vi "rsidr_core_global.vi"() -> ()   [LabVIEW 2020, in "Rohde&Schwarz RTx Oscilloscopes.lvlib"] (continued)
is defined by RSRTX_ATTR_HARDCOPY_SELECT_PRINTER attribute. The file name for storage is defined by RSRTX_ATTR_HARDCOPY_FILE_NAME attribute.\n\nAvailable Repeated Capabilities:\nNone\n\nRemote-control command(s):\nHCOPy[:IMMediate]"}, {"Level"=2, "Class Only"=FALSE, "Identifier"="RSRTX_ATTR_HARDCOPY_SELECT_PRINTER", "Descriptive Name"="Hardcopy Select Printer", "Data Type"=2, "Command"="SYST:COMM:PRIN:SEL", "Access"=2, "Range Table"="", "Read Callback"="", "Write Callback"="", "Supported Models"="", "Instrument Options"="", "Flags"=0, "Help"="Selects a configured printer. To determine which printers are installed, use the RSRTX_ATTR_HARDCOPY_GET_FIRST_PRINTER and RSRTX_ATTR_HARDCOPY_GET_NEXT_PRINTER attributes.\n\nAvailable Repeated Capabilities:\nNone\n\nRemote-control command(s):\nSYSTem:COMMunicate:PRINter:SELect"}, {"Level"=2, "Class Only"=FALSE, "Identifier"="RSRTX_ATTR_HARDCOPY_GET_FIRST_PRINTER", "Descriptive Name"="Hardcopy Get First Printer", "Data Type"=2, "Command"="SYST:COMM:PRIN:ENUM:FIRS?", "Access"=0, "Range Table"="", "Read Callback"="", "Write Callback"="", "Supported Models"="", "Instrument Options"="", "Flags"=0, "Help"="Queries the name of the first printer (in the list of printers) available.\nIf no printer is configured an empty string is output.\n\nAvailable Repeated Capabilities:\nNone\n\nRemote-control command(s):\nSYSTem:COMMunicate:PRINter:ENUMerate:FIRSt?"}, {"Level"=2, "Class Only"=FALSE, "Identifier"="RSRTX_ATTR_HARDCOPY_GET_NEXT_PRINTER", "Descriptive Name"="Hardcopy Get Next Printer", "Data Type"=2, "Command"="SYST:COMM:PRIN:ENUM:NEXT?", "Access"=0, "Range Table"="", "Read Callback"="", "Write Callback"="", "Supported Models"="", "Instrument Options"="", "Flags"=0, "Help"="Queries the name of the next printer installed. After all available printer names have been output, an empty string enclosed by quotation marks (&apos;&apos;) is output for the next query. Further queries are answered by a query error.\nThe RSRTX_ATTR_HARDCOPY_GET_FIRST_PRINTER attribute should be sent previously to return to the beginning of the printer list and query the name of the first printer.\n\nAvailable Repeated Capabilities:\nNone\n\nRemote-control command(s):\nSYSTem:COMMunicate:PRINter:ENUMerate[:NEXT]?"}, {"Level"=1, "Class Only"=TRUE, "Identifier"="", "Descriptive Name"="System", "Data Type"=0, "Command"="", "Access"=0, "Range Table"="", "Read Callback"="", "Write Callback"="", "Supported Models"="", "Instrument Options"="", "Flags"=0, "Help"="System attributes."}, {"Level"=2, "Class Only"=FALSE, "Identifier"="RSRTX_ATTR_DEVICE_MODE", "Descriptive Name"="Device Mode", "Data Type"=0, "Command"="DEV:MODE", "Access"=2, "Range Table"="RsRtx_rngDeviceMode", "Read Callback"="", "Write Callback"="", "Supported Models"="", "Instrument Options"="", "Flags"=0, "Help"="Configures the device mode.\n\nAvailable Repeated Capabilities:\nNone\n\nRemote-control command(s):\nDEVice:MODE"}, {"Level"=2, "Class Only"=FALSE, "Identifier"="RSRTX_ATTR_INTERFACE_SELECT", "Descriptive Name"="Interface Select", "Data Type"=0, "Command"="SYST:COMM:INT", "Access"=2, "Range Table"="RsRtx_rngInterface", "Read Callback"="", "Write Callback"="", "Supported Models"="", "Instrument Options"="", "Flags"=0, "Help"="Selects the interface for remote control and web browser access ( ETHernet only).\n\nAvailable Repeated Capabilities:\nNone\n\nRemote-control command(s):\nSYSTem:COMMunicate:INTerface[:SELect]"}, {"Level"=2, "Class Only"=FALSE, "Identifier"="RSRTX_ATTR_USB_CLASS", "Descriptive Name"="USB Class", "Data Type"=0, "Command"="SYST:COMM:INT:USB:CLAS", "Access"=2, "Range Table"="RsRtx_rngUSBClass", "Read Callback"="", "Write Callback"="", "Supported Models"="", "Instrument Options"="", "Flags"=0, "Help"="Selects the USB mode.\n\nAvailable Repeated Capabilities:\nNone\n\nRemote-control command(s):\nSYSTem:COMMunicate:INTerface:USB:CLASs"}, {"Level"=2, "Class Only"=FALSE, "Identifier"="RSRTX_ATTR_ETHERNET_DHCP", "Descriptive Name"="Ethernet DHCP", "Data Type"=3, "Command"="SYST:COMM:INT:ETH:DHCP", "Access"=2, "Range Table"="", "Read Callback"="", "Write Callback"="", "Supported Models"="", "Instrument Options"="", "Flags"=0, "Help"="Enables DHCP for automatic network parameter distribution.\n\nAvailable Repeated Capabilities:\nNone\n\nRemote-control command(s):\nSYSTem:COMMunicate:INTerface:ETHernet:DHCP"}, {"Level"=2, "Class Only"=FALSE, "Identifier"="RSRTX_ATTR_ETHERNET_IP_PORT", "Descriptive Name"="Ethernet IP Port", "Data Type"=0, "Command"="SYST:COMM:INT:ETH:IPP", "Access"=2, "Range Table"="RsRtx_rngEthernetIPPort", "Read Callback"="", "Write Callback"="", "Supported Models"="", "Instrument Options"="", "Flags"=0, "Help"="Specify the IP port number.\n\nAvailable Repeated Capabilities:\nNone\n\nRemote-control command(s):\nSYSTem:COMMunicate:INTerface:ETHernet:IPPort"}, {"Level"=2, "Class Only"=FALSE, "Identifier"="RSRTX_ATTR_ETHERNET_VXI11_PORT", "Descriptive Name"="Ethernet VXI11 Port", "Data Type"=0, "Command"="SYST:COMM:INT:ETH:VXIP", "Access"=2, "Range Table"="RsRtx_rng16BitRange", "Read Callback"="", "Write Callback"="", "Supported Models"="", "Instrument Options"="", "Flags"=0, "Help"="Returns or specifies the VXI-11 port number.\n\nAvailable Repeated Capabilities:\nNone\n\nRemote-control command(s):\nSYSTem:COMMunicate:INTerface:ETHernet:VXIPort"}, {"Level"=2, "Class Only"=FALSE, "Identifier"="RSRTX_ATTR_ETHERNET_HTTP_PORT", "Descriptive Name"="Ethernet HTTP Port", "Data Type"=0, "Command"="SYST:COMM:INT:ETH:HTTP", "Access"=2, "Range Table"="RsRtx_rng16BitRange", "Read Callback"="", "Write Callback"="", "Supported Models"="", "Instrument Options"="", "Flags"=0, "Help"="Returns or specifies the HTTP port number.\n\nAvailable Repeated Capabilities:\nNone\n\nRemote-control command(s):\nSYSTem:COMMunicate:INTerface:ETHernet:HTTPport"}, {"Level"=2, "Class Only"=FALSE, "Identifier"="RSRTX_ATTR_ETHERNET_TRANSFER", "Descriptive Name"="Ethernet Transfer", "Data Type"=0, "Command"="SYST:COMM:INT:ETH:TRAN", "Access"=2, "Range Table"="RsRtx_rngEthernetTransfer", "Read Callback"="", "Write Callback"="", "Supported Models"="", "Instrument Options"="", "Flags"=0, "Help"="Enables automatic transfer speed selection, or selects one of the predefined settings that corresponds to your network data rate.\n\nAvailable Repeated Capabilities:\nNone\n\nRemote-control command(s):\nSYSTem:COMMunicate:INTerface:ETHernet:TRANsfer"}, {"Level"=2, "Class Only"=FALSE, "Identifier"="RSRTX_ATTR_ETHERNET_MAC_ADDRESS", "Descriptive Name"="Ethernet MAC Address", "Data Type"=2, "Command"="SYST:COMM:INT:ETH:MAC?", "Access"=0, "Range Table"="", "Read Callback"="", "Write Callback"="", "Supported Models"="", "Instrument Options"="", "Flags"=0, "Help"="Returns the instrument&apos;s media access control address.\n\nAvailable Repeated Capabilities:\nNone\n\nRemote-control command(s):\nSYSTem:COMMunicate:INTerface:ETHernet:MACaddress?"}, {"Level"=2, "Class Only"=FALSE, "Identifier"="RSRTX_ATTR_PRESET_EDUCATION", "Descriptive Name"="Preset Education", "Data Type"=4, "Command"="SYST:EDUC:PRES", "Access"=1, "Range Table"="", "Read Callback"="", "Write Callback"="", "Supported Models"="", "Instrument Options"="", "Flags"=0, "Help"="Deletes the password of the education mode.\n\nAvailable Repeated Capabilities:\nNone\n\nRemote-control command(s):\nSYSTem:EDUCation:PRESet"}, {"Level"=2, "Class Only"=FALSE, "Identifier"="RSRTX_ATTR_DEVICE_FOOTPRINT", "Descriptive Name"="Device Footprint", "Data Type"=2, "Command"="SYST:DFPR?", "Access"=0, "Range Table"="", "Read Callback"="", "Write Callback"="", "Supported Models"="", "Instrument Options"="", "Flags"=0, "Help"="Returns the device footprint of the instrument. The device footprint contains the configuration of the instrument, installed modules, installed software and software licenses. This information is written in the device footprint xml file might be useful in case of maintenance or support request.\n\nAvailable Repeated Capabilities:\nNone\n\nRemote-control command(s):\nSYSTem:DFPRint?"}, {"Level"=1, "Class Only"=TRUE, "Identifier"="", "Descriptive Name"="Utility Functions", "Data Type"=0, "Command"="", "Access"=0, "Range Table"="", "Read Callback"="", "Write Callback"="", "Supported Models"="", "Instrument Options"="", "Flags"=0, "Help"="This subsystem contains functions for Utility Functions."}, {"Level"=2, "Class Only"=FALSE, "Identifier"="RSRTX_ATTR_SYSTEM_PRESET", "Descriptive Name"="System Preset", "Data Type"=4, "Command"="SYST:PRES", "Access"=1, "Range Table"="", "Read Callback"="", "Write Callback"="", "Supported Models"="", "Instrument Options"="", "Flags"=0, "Help"="Presets all parameters.\n\nAvailable Repeated Capabilities:\nNone\n\nRemote-control command(s):\nSYSTem:PRESet"}, {"Level"=2, "Class Only"=FALSE, "Identifier"="RSRTX_ATTR_CALIBRATION", "Descriptive Name"="Calibration", "Data Type"=0, "Command"="*CAL?", "Access"=0, "Range Table"="", "Read Callback"="", "Write Callback"="", "Supported Models"="", "Instrument Options"="", "Flags"=0, "Help"="Initiates a calibration of the instrument and subsequently queries the calibration status. Responses > 0 indicate errors.\n\nAvailable Repeated Capabilities:\nNone\n\nRemote-control command(s):\n*CAL?"}, {"Level"=2, "Class Only"=FALSE, "Identifier"="RSRTX_ATTR_SELF_TEST_QUERY", "Descriptive Name"="Self-Test Query", "Data Type"=0, "Command"="*TST?", "Access"=0, "Range Table"="", "Read Callback"="", "Write Callback"="", "Supported Models"="", "Instrument Options"="", "Flags"=1, "Help"="Triggers selftests of the instrument and returns an error code in decimal form (see Service Manual supplied with the instrument). 0 indicates no errors occured.\n\nAvailable Repeated Capabilities:\nNone\n\nRemote-control command(s):\n*TST?"}, {"Level"=2, "Class Only"=FALSE, "Identifier"="RSRTX_ATTR_SYSTEM_ERROR", "Descriptive Name"="System Error", "Data Type"=2, "Command"="SYST:ERR?", "Access"=0, "Range Table"="", "Read Callback"="", "Write Callback"="", "Supported Models"="", "Instrument Options"="", "Flags"=0, "Help"="Queries error from error queue.\n\nAvailable Repeated Capabilities:\nNone\n\nRemote-control command(s):\nSYSTem:ERRor:[NEXT]?"}, {"Level"=2, "Class Only"=FALSE, "Identifier"="RSRTX_ATTR_SYST_ERR_LIST", "Descriptive Name"="System Error List", "Data Type"=2, "Command"="SYST:ERR:ALL?", "Access"=0, "Range Table"="", "Read Callback"="", "Write Callback"="", "Supported Models"="", "Instrument Options"="", "Flags"=0, "Help"="Returns the error message string read from the instrument&apos;s error message queue.\n\nAvailable Repeated Capabilities:\nNone\n\nRemote-control command(s):\nSYSTem:ERRor:ALL?"}, {"Level"=2, "Class Only"=FALSE, "Identifier"="RSRTX_ATTR_INSTRUMENT_NAME", "Descriptive Name"="Instrument Name", "Data Type"=2, "Command"="SYST:NAME", "Access"=2, "Range Table"="", "Read Callback"="", "Write Callback"="", "Supported Models"="", "Instrument Options"="", "Flags"=0, "Help"="Defines an instrument name (String with max. 20 characters).\n\nAvailable Repeated Capabilities:\nNone\n\nRemote-control command(s):\nSYSTem:NAME"}, {"Level"=2, "Class Only"=FALSE, "Identifier"="RSRTX_ATTR_RESET_STATUS_REGISTER", "Descriptive Name"="Reset Status Register", "Data Type"=4, "Command"="STAT:PRES", "Access"=1, "Range Table"="", "Read Callback"="", "Write Callback"="", "Supported Models"="", "Instrument Options"="", "Flags"=0, "Help"="Resets all STATUS:QUESTIONALBLE registers.\n\nAvailable Repeated Capabilities:\nNone\n\nRemote-control command(s):\nSTATus:PRESet"}, {"Level"=2, "Class Only"=FALSE, "Identifier"="RSRTX_ATTR_SELF_ALIGNMENT", "Descriptive Name"="Self Alignment", "Data Type"=4, "Command"="CAL", "Access"=1, "Range Table"="", "Read Callback"="", "Write Callback"="", "Supported Models"="", "Instrument Options"="", "Flags"=0, "Help"="Executes an internal self-alignment of the instrument.\n\nAvailable Repeated Capabilities:\nNone\n\nRemote-control command(s):\nCALibration"}, {"Level"=2, "Class Only"=FALSE, "Identifier"="RSRTX_ATTR_SELF_ALIGNMENT_STATE", "Descriptive Name"="Self Alignment State", "Data Type"=0, "Command"="CAL:STAT?", "Access"=0, "Range Table"="rsrtx_rngSelfAlignmentState", "Read Callback"="", "Write Callback"="", "Supported Models"="", "Instrument Options"="", "Flags"=0, "Help"="Returns the overall state of the self-alignment.\n\nAvailable Repeated Capabilities:\nNone\n\nRemote-control command(s):\nCALibration:STATe?"}, {"Level"=2, "Class Only"=FALSE, "Identifier"="RSRTX_ATTR_QUERY_OPC", "Descriptive Name"="Query OPC", "Data Type"=0, "Command"="*OPC?", "Access"=0, "Range Table"="", "Read Callback"="", "Write Callback"="", "Supported Models"="", "Instrument Options"="", "Flags"=0, "Help"="Queries the OPC.\n\nAvailable Repeated Capabilities:\nNone\n\nRemote-control command(s):\n*OPC?"}, {"Level"=2, "Class Only"=FALSE, "Identifier"="RSRTX_ATTR_PROCESS_ALL_PREVIOUS_COMMANDS", "Descriptive Name"="Process All Previous Commands", "Data Type"=4, "Command"="*WAI", "Access"=1, "Range Table"="", "Read Callback"="", "Write Callback"="", "Supported Models"="", "Instrument Options"="", "Flags"=2, "Help"="Stops further command processing until all commands sent before *WAI have been executed.\n\nAvailable Repeated Capabilities:\nNone\n\nRemote-control command(s):\n*WAI"}, {"Level"=2, "Class Only"=TRUE, "Identifier"="", "Descriptive Name"="Sound", "Data Type"=0, "Command"="", "Access"=0, "Range Table"="", "Read Callback"="", "Write Callback"="", "Supported Models"="", "Instrument Options"="", "Flags"=0, "Help"="Additional Sound Attributes."}, {"Level"=3, "Class Only"=FALSE, "Identifier"="RSRTX_ATTR_SOUND_ENABLED", "Descriptive Name"="Sound Enabled", "Data Type"=3, "Command"="SYST:BEEP:CONT:STAT", "Access"=2, "Range Table"="", "Read Callback"="", "Write Callback"="", "Supported Models"="", "Instrument Options"="", "Flags"=0, "Help"="Enables or diables a sound for general control events, e.g. reaching the rotary encoder end or changing the measuring mode in the Automeasure menu.\n\nAvailable Repeated Capabilities:\nNone\n\nRemote-control command(s):\nSYSTem:BEEPer:CONTrol:STATe"}, {"Level"=3, "Class Only"=FALSE, "Identifier"="RSRTX_ATTR_SOUND_ERROR_ENABLED", "Descriptive Name"="Sound Error Enabled", "Data Type"=3, "Command"="SYST:BEEP:ERR:STAT", "Access"=2, "Range Table"="", "Read Callback"="", "Write Callback"="", "Supported Models"="", "Instrument Options"="", "Flags"=0, "Help"="Enables or disables the beep if an error occurs.\n\nAvailable Repeated Capabilities:\nNone\n\nRemote-control command(s):\nSYSTem:BEEPer:ERRor:STATe"}, {"Level"=3, "Class Only"=FALSE, "Identifier"="RSRTX_ATTR_SOUND_TRIGGER_ENABLED", "Descriptive Name"="Sound Trigger Enabled", "Data Type"=3, "Command"="SYST:BEEP:TRIG:STAT", "Access"=2, "Range Table"="", "Read Callback"="", "Write Callback"="", "Supported Models"="", "Instrument Options"="", "Flags"=0, "Help"="Enables or disables the beep if a trigger occurs.\n\nAvailable Repeated Capabilities:\nNone\n\nRemote-control command(s):\nSYSTem:BEEPer:TRIG:STATe"}, {"Level"=3, "Class Only"=FALSE, "Identifier"="RSRTX_ATTR_SOUND_GENERATE", "Descriptive Name"="Sound Generate", "Data Type"=4, "Command"="SYST:BEEP", "Access"=1, "Range Table"="", "Read Callback"="", "Write Callback"="", "Supported Models"="", "Instrument Options"="", "Flags"=0, "Help"="Generates an immediate beep.\n\nAvailable Repeated Capabilities:\nNone\n\nRemote-control command(s):\nSYSTem:BEEPer[:IMMediate]"}, {"Level"=2, "Class Only"=TRUE, "Identifier"="", "Descriptive Name"="Status Register", "Data Type"=0, "Command"="", "Access"=0, "Range Table"="", "Read Callback"="", "Write Callback"="", "Supported Models"="", "Instrument Options"="", "Flags"=0, "Help"="Configures the status reporting system."}, {"Level"=3, "Class Only"=TRUE, "Identifier"="", "Descriptive Name"="Operation", "Data Type"=0, "Command"="", "Access"=0, "Range Table"="", "Read Callback"="", "Write Callback"="", "Supported Models"="", "Instrument Options"="", "Flags"=0, "Help"="Configures the operation status reporting system."}, {"Level"=4, "Class Only"=FALSE, "Identifier"="RSRTX_ATTR_OPERATION_CONDITION", "Descriptive Name"="Operation Condition", "Data Type"=0, "Command"="STAT:OPER:COND?", "Access"=0, "Range Table"="", "Read Callback"="", "Write Callback"="", "Supported Models"="", "Instrument Options"="", "Flags"=0, "Help"="Sets the status reporting system Operation Condition.\n\nNote:\n(1) For detailed description of Status Reporting System see also operating manual.\n\nAvailable Repeated Capabilities:\nNone\n\nRemote-control command(s):\nSTATus:OPERation:CONDition?"}, {"Level"=4, "Class Only"=FALSE, "Identifier"="RSRTX_ATTR_OPERATION_ENABLE", "Descriptive Name"="Operation Enable", "Data Type"=0, "Command"="STAT:OPER:ENAB", "Access"=2, "Range Table"="", "Read Callback"="", "Write Callback"="", "Supported Models"="", "Instrument Options"="", "Flags"=0, "Help"="Sets the status reporting system Operation Enable.\n\nNote:\n(1) For detailed description of Status Reporting System see also operating manual.\n\nAvailable Repeated Capabilities:\nNone\n\nRemote-control command(s):\nSTATus:OPERation:ENABle"}, {"Level"=4, "Class Only"=FALSE, "Identifier"="RSRTX_ATTR_OPERATION_N_TRANSITION", "Descriptive Name"="Operation N Transition", "Data Type"=0, "Command"="STAT:OPER:NTR", "Access"=2, "Range Table"="", "Read Callback"="", "Write Callback"="", "Supported Models"="", "Instrument Options"="", "Flags"=0, "Help"="Sets the status reporting system Operation N Transition.\n\nNote:\n(1) For detailed description of Status Reporting System see also operating manual.\n\nAvailable Repeated Capabilities:\nNone\n\nRemote-control command(s):\nSTATus:OPERation:NTRansition"}, {"Level"=4, "Class Only"=FALSE, "Identifier"="RSRTX_ATTR_OPERATION_P_TRANSITION", "Descriptive Name"="Operation P Transition", "Data Type"=0, "Command"="STAT:OPER:PTR", "Access"=2, "Range Table"="", "Read Callback"="", "Write Callback"="", "Supported Models"="", "Instrument Options"="", "Flags"=0, "Help"="Sets the status reporting system Operation P Transition.\n\nNote:\n(1) For detailed description of Status Reporting System see also operating manual.\n\nAvailable Repeated Capabilities:\nNone\n\nRemote-control command(s):\nSTATus:OPERation:PTRansition"}, {"Level"=4, "Class Only"=FALSE, "Identifier"="RSRTX_ATTR_OPERATION_EVENT", "Descriptive Name"="Operation Event", "Data Type"=0, "Command"="STAT:OPER?", "Access"=0, "Range Table"="", "Read Callback"="", "Write Callback"="", "Supported Models"="", "Instrument Options"="", "Flags"=0, "Help"="Sets the status reporting system Operation Event.\n\nNote:\n(1) For detailed description of Status Reporting System see also operating manual.\n\nAvailable Repeated Capabilities:\nNone\n\nRemote-control command(s):\nSTATus:OPERation[:EVENt]?"}, {"Level"=3, "Class Only"=TRUE, "Identifier"="", "Descriptive Name"="Questionable", "Data Type"=0, "Command"="", "Access"=0, "Range Table"="", "Read Callback"="", "Write Callback"="", "Supported Models"="", "Instrument Options"="", "Flags"=0, "Help"="Configures the questionable status reporting system."}, {"Level"=4, "Class Only"=FALSE, "Identifier"="RSRTX_ATTR_QUESTIONABLE_CONDITION", "Descriptive Name"="Questionable Condition", "Data Type"=0, "Command"="STAT:QUES:COND?", "Access"=0, "Range Table"="RsRtx_rng16BitRange", "Read Callback"="", "Write Callback"="", "Supported Models"="", "Instrument Options"="", "Flags"=0, "Help"="Sets the status reporting system Questionable Condition.\n\nNote:\n(1) For detailed description of Status Reporting System see also operating manual.\n\nAvailable Repeated Capabilities:\nNone\n\nRemote-control command(s):\nSTATus:QUEStionable:CONDition?"}, {"Level"=4, "Class Only"=FALSE, "Identifier"="RSRTX_ATTR_QUESTIONABLE_ENABLE", "Descriptive Name"="Questionable Enable", "Data Type"=0, "Command"="STAT:QUES:ENAB", "Access"=2, "Range Table"="RsRtx_rng16BitRange", "Read Callback"="", "Write Callback"="", "Supported Models"="", "Instrument Options"="", "Flags"=0, "Help"="Sets the status reporting system Questionable Enable.\n\nNote:\n(1) For detailed description of Status Reporting System see also operating manual.\n\nAvailable Repeated Capabilities:\nNone\n\nRemote-control command(s):\nSTATus:QUEStionable:ENABle"}, {"Level"=4, "Class Only"=FALSE, "Identifier"="RSRTX_ATTR_QUESTIONABLE_N_TRANSITION", "Descriptive Name"="Questionable N Transition", "Data Type"=0, "Command"="STAT:QUES:NTR", "Access"=2, "Range Table"="RsRtx_rng16BitRange", "Read Callback"="", "Write Callback"="", "Supported Models"="", "Instrument Options"="", "Flags"=0, "Help"="Sets the status reporting system Questionable N Transition.\n\nNote:\n(1) For detailed description of Status Reporting System see also operating manual.\n\nAvailable Repeated Capabilities:\nNone\n\nRemote-control command(s):\nSTATus:QUEStionable:NTRansition"}, {"Level"=4, "Class Only"=FALSE, "Identifier"="RSRTX_ATTR_QUESTIONABLE_P_TRANSITION", "Descriptive Name"="Questionable P Transition", "Data Type"=0, "Command"="STAT:QUES:PTR", "Access"=2, "Range Table"="RsRtx_rng16BitRange", "Read Callback"="", "Write Callback"="", "Supported Models"="", "Instrument Options"="", "Flags"=0, "Help"="Sets the status reporting system Questionable P Transition.\n\nNote:\n(1) For detailed description of Status Reporting System see also operating manual.\n\nAvailable Repeated Capabilities:\nNone\n\nRemote-control command(s):\nSTATus:QUEStionable:PTRansition"}, {"Level"=4, "Class Only"=FALSE, "Identifier"="RSRTX_ATTR_QUESTIONABLE_EVENT", "Descriptive Name"="Questionable Event", "Data Type"=0, "Command"="STAT:QUES?", "Access"=0, "Range Table"="RsRtx_rng16BitRange", "Read Callback"="", "Write Callback"="", "Supported Models"="", "Instrument Options"="", "Flags"=0, "Help"="Sets the status reporting system Questionable Event.\n\nNote:\n(1) For detailed description of Status Reporting System see also operating manual.\n\nAvailable Repeated Capabilities:\nNone\n\nRemote-control command(s):\nSTATus:QUEStionable[:EVENt]?"}, {"Level"=4, "Class Only"=TRUE, "Identifier"="", "Descriptive Name"="Channel Overload", "Data Type"=0, "Command"="", "Access"=0, "Range Table"="", "Read Callback"="", "Write Callback"="", "Supported Models"="", "Instrument Options"="", "Flags"=0, "Help"="Configures the questionable channel overload status reporting system."}, {"Level"=5, "Class Only"=FALSE, "Identifier"="RSRTX_ATTR_QUESTIONABLE_CHANNEL_OVERLOAD_CONDITION", "Descriptive Name"="Questionable Channel Overload Condition", "Data Type"=0, "Command"="STAT:QUES:COV:COND?", "Access"=0, "Range Table"="RsRtx_rng16BitRange", "Read Callback"="", "Write Callback"="", "Supported Models"="", "Instrument Options"="", "Flags"=0, "Help"="Sets the status reporting system Questionable Channel Overload Condition.\n\nNote:\n(1) For detailed description of Status Reporting System see also operating manual.\n\nAvailable Repeated Capabilities:\nNone\n\nRemote-control command(s):\nSTATus:QUEStionable:COVerload:CONDition?"}, {"Level"=5, "Class Only"=FALSE, "Identifier"="RSRTX_ATTR_QUESTIONABLE_CHANNEL_OVERLOAD_ENABLE", "Descriptive Name"="Questionable Channel Overload Enable", "Data Type"=0, "Command"="STAT:QUES:COV:ENAB", "Access"=2, "Range Table"="RsRtx_rng16BitRange", "Read Callback"="", "Write Callback"="", "Supported Models"="", "Instrument Options"="", "Flags"=0, "Help"="Sets the status reporting system Questionable Channel Overload Enable.\n\nNote:\n(1) For detailed description of Status Reporting System see also operating manual.\n\nAvailable Repeated Capabilities:\nNone\n\nRemote-control command(s):\nSTATus:QUEStionable:COVerload:ENABle"}, {"Level"=5, "Class Only"=FALSE, "Identifier"="RSRTX_ATTR_QUESTIONABLE_CHANNEL_OVERLOAD_N_TRANSITION", "Descriptive Name"="Questionable Channel Overload N Transition", "Data Type"=0, "Command"="STAT:QUES:COV:NTR", "Access"=2, "Range Table"="RsRtx_rng16BitRange", "Read Callback"="", "Write Callback"="", "Supported Models"="", "Instrument Options"="", "Flags"=0, "Help"="Sets the status reporting system Questionable Channel Overload N Transition.\n\nNote:\n(1) For detailed description of Status Reporting System see also operating manual.\n\nAvailable Repeated Capabilities:\nNone\n\nRemote-control command(s):\nSTATus:QUEStionable:COVerload:NTRansition"}, {"Level"=5, "Class Only"=FALSE, "Identifier"="RSRTX_ATTR_QUESTIONABLE_CHANNEL_OVERLOAD_P_TRANSITION", "Descriptive Name"="Questionable Channel Overload P Transition", "Data Type"=0, "Command"="STAT:QUES:COV:PTR", "Access"=2, "Range Table"="RsRtx_rng16BitRange", "Read Callback"="", "Write Callback"="", "Supported Models"="", "Instrument Options"="", "Flags"=0, "Help"="Sets the status reporting system Questionable Channel Overload P Transition.\n\nNote:\n(1) For detailed description of Status Reporting System see also operating manual.\n\nAvailable Repeated Capabilities:\nNone\n\nRemote-control command(s):\nSTATus:QUEStionable:COVerload:PTRansition"}, {"Level"=5, "Class Only"=FALSE, "Identifier"="RSRTX_ATTR_QUESTIONABLE_CHANNEL_OVERLOAD_EVENT", "Descriptive Name"="Questionable Channel Overload Event", "Data Type"=0, "Command"="STAT:QUES:COV?", "Access"=0, "Range Table"="RsRtx_rng16BitRange", "Read Callback"="", "Write Callback"="", "Supported Models"="", "Instrument Options"="", "Flags"=0, "Help"="Sets the status reporting system Questionable Channel Overload Event.\n\nNote:\n(1) For detailed description of Status Reporting System see also operating manual.\n\nAvailable Repeated Capabilities:\nNone\n\nRemote-control command(s):\nSTATus:QUEStionable:COVerload[:EVENt]?"}, {"Level"=4, "Class Only"=TRUE, "Identifier"="", "Descriptive Name"="Limit", "Data Type"=0, "Command"="", "Access"=0, "Range Table"="", "Read Callback"="", "Write Callback"="", "Supported Models"="", "Instrument Options"="", "Flags"=0, "Help"="Configures the questionable limit status reporting system."}, {"Level"=5, "Class Only"=FALSE, "Identifier"="RSRTX_ATTR_QUESTIONABLE_LIMIT_CONDITION", "Descriptive Name"="Questionable Limit Condition", "Data Type"=0, "Command"="STAT:QUES:LIM:COND?", "Access"=0, "Range Table"="RsRtx_rng16BitRange", "Read Callback"="", "Write Callback"="", "Supported Models"="", "Instrument Options"="", "Flags"=0, "Help"="Sets the status reporting system Questionable Limit Condition.\n\nNote:\n(1) For detailed description of Status Reporting System see also operating manual.\n\nAvailable Repeated Capabilities:\nNone\n\nRemote-control command(s):\nSTATus:QUEStionable:LIMit:CONDition?"}, {"Level"=5, "Class Only"=FALSE, "Identifier"="RSRTX_ATTR_QUESTIONABLE_LIMIT_ENABLE", "Descriptive Name"="Questionable Limit Enable", "Data Type"=0, "Command"="STAT:QUES:LIM:ENAB", "Access"=2, "Range Table"="RsRtx_rng16BitRange", "Read Callback"="", "Write Callback"="", "Supported Models"="", "Instrument Options"="", "Flags"=0, "Help"="Sets the status reporting system Questionable Limit Enable.\n\nNote:\n(1) For detailed description of Status Reporting System see also operating manual.\n\nAvailable Repeated Capabilities:\nNone\n\nRemote-control command(s):\nSTATus:QUEStionable:LIMit:ENABle"}, {"Level"=5, "Class Only"=FALSE, "Identifier"="RSRTX_ATTR_QUESTIONABLE_LIMIT_N_TRANSITION", "Descriptive Name"="Questionable Limit N Transition", "Data Type"=0, "Command"="STAT:QUES:LIM:NTR", "Access"=2, "Range Table"="RsRtx_rng16BitRange", "Read Callback"="", "Write Callback"="", "Supported Models"="", "Instrument Options"="", "Flags"=0, "Help"="Sets the status reporting system Questionable Limit N Transition.\n\nNote:\n(1) For detailed description of Status Reporting System see also operating manual.\n\nAvailable Repeated Capabilities:\nNone\n\nRemote-control command(s):\nSTATus:QUEStionable:LIMit:NTRansition"}, {"Level"=5, "Class Only"=FALSE, "Identifier"="RSRTX_ATTR_QUESTIONABLE_LIMIT_P_TRANSITION", "Descriptive Name"="Questionable Limit P Transition", "Data Type"=0, "Command"="STAT:QUES:LIM:PTR", "Access"=2, "Range Table"="RsRtx_rng16BitRange", "Read Callback"="", "Write Callback"="", "Supported Models"="", "Instrument Options"="", "Flags"=0, "Help"="Sets the status reporting system Questionable Limit P Transition.\n\nNote:\n(1) For detailed description of Status Reporting System see also operating manual.\n\nAvailable Repeated Capabilities:\nNone\n\nRemote-control command(s):\nSTATus:QUEStionable:LIMit:PTRansition"}, {"Level"=5, "Class Only"=FALSE, "Identifier"="RSRTX_ATTR_QUESTIONABLE_LIMIT_EVENT", "Descriptive Name"="Questionable Limit Event", "Data Type"=0, "Command"="STAT:QUES:LIM?", "Access"=0, "Range Table"="RsRtx_rng16BitRange", "Read Callback"="", "Write Callback"="", "Supported Models"="", "Instrument Options"="", "Flags"=0, "Help"="Sets the status reporting system Questionable Limit Event.\n\nNote:\n(1) For detailed description of Status Reporting System see also operating manual.\n\nAvailable Repeated Capabilities:\nNone\n\nRemote-control command(s):\nSTATus:QUEStionable:LIMit[:EVENt]?"}, {"Level"=4, "Class Only"=TRUE, "Identifier"="", "Descriptive Name"="Mask", "Data Type"=0, "Command"="", "Access"=0, "Range Table"="", "Read Callback"="", "Write Callback"="", "Supported Models"="", "Instrument Options"="", "Flags"=0, "Help"="Configures the questionable mask status reporting system."}, {"Level"=5, "Class Only"=FALSE, "Identifier"="RSRTX_ATTR_QUESTIONABLE_MASK_CONDITION", "Descriptive Name"="Questionable Mask Condition", "Data Type"=0, "Command"="STAT:QUES:MASK:COND?", "Access"=0, "Range Table"="RsRtx_rng16BitRange", "Read Callback"="", "Write Callback"="", "Supported Models"="", "Instrument Options"="", "Flags"=0, "Help"="Sets the status reporting system Questionable Mask Condition.\n\nNote:\n(1) For detailed description of Status Reporting System see also operating manual.\n\nAvailable Repeated Capabilities:\nNone\n\nRemote-control command(s):\nSTATus:QUEStionable:MASK:CONDition?"}, {"Level"=5, "Class Only"=FALSE, "Identifier"="RSRTX_ATTR_QUESTIONABLE_MASK_ENABLE", "Descriptive Name"="Questionable Mask Enable", "Data Type"=0, "Command"="STAT:QUES:MASK:ENAB", "Access"=2, "Range Table"="RsRtx_rng16BitRange", "Read Callback"="", "Write Callback"="", "Supported Models"="", "Instrument Options"="", "Flags"=0, "Help"="Sets the status reporting system Questionable Mask Enable.\n\nNote:\n(1) For detailed description of Status Reporting System see also operating manual.\n\nAvailable Repeated Capabilities:\nNone\n\nRemote-control command(s):\nSTATus:QUEStionable:MASK:ENABle"}, {"Level"=5, "Class Only"=FALSE, "Identifier"="RSRTX_ATTR_QUESTIONABLE_MASK_N_TRANSITION", "Descriptive Name"="Questionable Mask N Transition", "Data Type"=0, "Command"="STAT:QUES:MASK:NTR", "Access"=2, "Range Table"="RsRtx_rng16BitRange", "Read Callback"="", "Write Callback"="", "Supported Models"="", "Instrument Options"="", "Flags"=0, "Help"="Sets the status reporting system Questionable Mask N Transition.\n\nNote:\n(1) For detailed description of Status Reporting System see also operating manual.\n\nAvailable Repeated Capabilities:\nNone\n\nRemote-control command(s):\nSTATus:QUEStionable:MASK:NTRansition"}, {"Level"=5, "Class Only"=FALSE, "Identifier"="RSRTX_ATTR_QUESTIONABLE_MASK_P_TRANSITION", "Descriptive Name"="Questionable Mask P Transition", "Data Type"=0, "Command"="STAT:QUES:MASK:PTR", "Access"=2, "Range Table"="RsRtx_rng16BitRange", "Read Callback"="", "Write Callback"="", "Supported Models"="", "Instrument Options"="", "Flags"=0, "Help"="Sets the status reporting system Questionable Mask P Transition.\n\nNote:\n(1) For detailed description of Status Reporting System see also operating manual.\n\nAvailable Repeated Capabilities:\nNone\n\nRemote-control command(s):\nSTATus:QUEStionable:MASK:PTRansition"}, {"Level"=5, "Class Only"=FALSE, "Identifier"="RSRTX_ATTR_QUESTIONABLE_MASK_EVENT", "Descriptive Name"="Questionable Mask Event", "Data Type"=0, "Command"="STAT:QUES:MASK?", "Access"=0, "Range Table"="RsRtx_rng16BitRange", "Read Callback"="", "Write Callback"="", "Supported Models"="", "Instrument Options"="", "Flags"=0, "Help"="Sets the status reporting system Questionable Mask Event.\n\nNote:\n(1) For detailed description of Status Reporting System see also operating manual.\n\nAvailable Repeated Capabilities:\nNone\n\nRemote-control command(s):\nSTATus:QUEStionable:MASK[:EVENt]?"}, {"Level"=4, "Class Only"=TRUE, "Identifier"="", "Descriptive Name"="ADC State", "Data Type"=0, "Command"="", "Access"=0, "Range Table"="", "Read Callback"="", "Write Callback"="", "Supported Models"="", "Instrument Options"="", "Flags"=0, "Help"="Configures the questionable ADC overflow reporting system."}, {"Level"=5, "Class Only"=FALSE, "Identifier"="RSRTX_ATTR_QUESTIONABLE_ADC_STATE_CONDITION", "Descriptive Name"="Questionable ADC State Condition", "Data Type"=0, "Command"="STAT:QUES:ADCS:COND?", "Access"=0, "Range Table"="", "Read Callback"="", "Write Callback"="", "Supported Models"="", "Instrument Options"="", "Flags"=0, "Help"="Returns the contents of the CONDition part of the status register to check for questionable instrument or measurement states. Reading the CONDition registers does not delete the contents.\n\nAvailable Repeated Capabilities:\nNone\n\nRemote-control command(s):\nSTATus:QUEStionable:ADCState:CONDition?"}, {"Level"=5, "Class Only"=FALSE, "Identifier"="RSRTX_ATTR_QUESTIONABLE_ADC_STATE_ENABLE", "Descriptive Name"="Questionable ADC State Enable", "Data Type"=0, "Command"="STAT:QUES:ADCS:ENAB", "Access"=2, "Range Table"="RsRtx_rng16BitRange", "Read Callback"="", "Write Callback"="", "Supported Models"="", "Instrument Options"="", "Flags"=0, "Help"="Sets the ENABle part that allows true conditions in the EVENt part to be reported in the summary bit. If a bit is set to 1 in the enable part and its associated event bit transitions to true, a positive transition occurs in the summary bit and is reported to the next higher level.\n\nAvailable Repeated Capabilities:\nNone\n\nRemote-control command(s):\nSTATus:QUEStionable:ADCState:ENABle"}, {"Level"=5, "Class Only"=FALSE, "Identifier"="RSRTX_ATTR_QUESTIONABLE_ADC_STATE_N_TRANSITION", "Descriptive Name"="Questionable ADC State N Transition", "Data Type"=0, "Command"="STAT:QUES:ADCS:NTR", "Access"=2, "Range Table"="RsRtx_rng16BitRange", "Read Callback"="", "Write Callback"="", "Supported Models"="", "Instrument Options"="", "Flags"=0, "Help"="Sets the negative transition filter. If a bit is set, a 1 to 0 transition in the corresponding bit of the condition register causes a 1 to be written in the corresponding bit of the event register.\n\nAvailable Repeated Capabilities:\nNone\n\nRemote-control command(s):\nSTATus:QUEStionable:ADCState:NTRansition"}, {"Level"=5, "Class Only"=FALSE, "Identifier"="RSRTX_ATTR_QUESTIONABLE_ADC_STATE_P_TRANSITION", "Descriptive Name"="Questionable ADC State P Transition", "Data Type"=0, "Command"="STAT:QUES:ADCS:PTR", "Access"=2, "Range Table"="RsRtx_rng16BitRange", "Read Callback"="", "Write Callback"="", "Supported Models"="", "Instrument Options"="", "Flags"=0, "Help"="Sets the positive transition filter. If a bit is set, a 0 to 1 transition in the corresponding bit of the condition register causes a 1 to be written in the corresponding bit of the event register.\n\nAvailable Repeated Capabilities:\nNone\n\nRemote-control command(s):\nSTATus:QUEStionable:ADCState:PTRansition"}, {"Level"=5, "Class Only"=FALSE, "Identifier"="RSRTX_ATTR_QUESTIONABLE_ADC_STATE_EVENT", "Descriptive Name"="Questionable ADC State Event", "Data Type"=0, "Command"="STAT:QUES:ADCS?", "Access"=0, "Range Table"="RsRtx_rng16BitRange", "Read Callback"="", "Write Callback"="", "Supported Models"="", "Instrument Options"="", "Flags"=0, "Help"="Returns the contents of the EVENt part of the status register to check whether an event has occurred since the last reading. Reading an EVENt register deletes its contents.\n\nAvailable Repeated Capabilities:\nNone\n\nRemote-control command(s):\nSTATus:QUEStionable:ADCState[:EVENt]?"}] {"Flags" format="%08b"; "Access" items=["Read Only", "Write Only", "Read/Write"]; "Data Type" items=["Integer 32", "Double", "String", "Boolean", "None", "Integer 64", "RawString"]}
  in  "Supported Models":string[](array[string])=["RTB", "RTM", "RTA"]
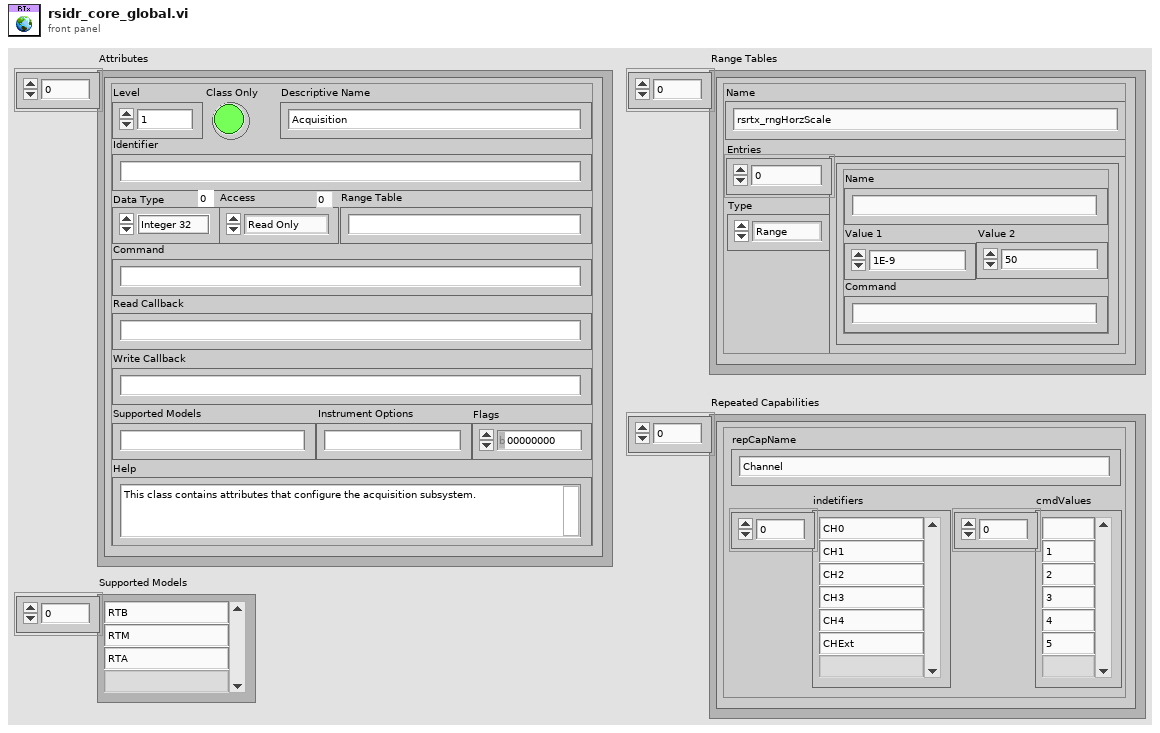
[diagram p1: front panel]
types:
  T1 = typedef "Rohde&Schwarz RTx Oscilloscopes.lvlib/rsidr_core.lvlib/type_Input_Format_RepCap.ctl" = cluster{"repCapName":string, "indetifiers":string[], "cmdValues":string[]}
  T2 = typedef "Rohde&Schwarz RTx Oscilloscopes.lvlib/rsidr_core.lvlib/type_Input_Format_RangeTable.ctl" = cluster{"Type":u16, "Name":string, "Entries":cluster{"Name":string, "Value 1":dbl, "Value 2":dbl, "Command":string}[]}
  T3 = typedef "Rohde&Schwarz RTx Oscilloscopes.lvlib/rsidr_core.lvlib/type_Input_Format_Attribute.ctl" = cluster{"Level":i32, "Class Only":bool, "Identifier":string, "Descriptive Name":string, "Data Type":u16, "Command":string, "Access":u16, "Range Table":string, "Read Callback":string, "Write Callback":string, "Supported Models":string, "Instrument Options":string, "Flags":i32, "Help":string}
diagram:
